vi "Close.vi"(8 "error in":errorcluster, 11 "Climate Chamber in":refnum<class "Climate Chamber.lvclass">) -> (0 "error out":errorcluster, 3 "Climate Chamber out":refnum<class "Climate Chamber.lvclass">)   [LabVIEW 2023, in "Climate Chamber.lvclass"]
uses:
  Climate Chamber.lvclass
  Climate Chamber.lvclass/Climate Chamber.ctl
  Low Level Capabilities/OnOff/OnOff.lvclass
  Low Level Capabilities/Temperature/Temperature Setpoint/Temperature Setpoint.lvclass
  Low Level Capabilities/Temperature/Temperature Actual Value/Temperature Actual Value.lvclass
  Low Level Capabilities/Error/Error.lvclass
  Low Level Capabilities/Temperature/Temperature Gradient/Temperature Gradient.lvclass
  Low Level Capabilities/Temperature/Temperature Limit/Temperature Limit.lvclass
  Low Level Capabilities/Humidity/Humidity Setpoint/Humidity Setpoint.lvclass
  Low Level Capabilities/Humidity/Humidity Limit/Humidity Limit.lvclass
  Low Level Capabilities/Humidity/Humidity Gradient/Humidity Gradient.lvclass
  Low Level Capabilities/Humidity/Humidity Actual Value/Humidity Actual Value.lvclass
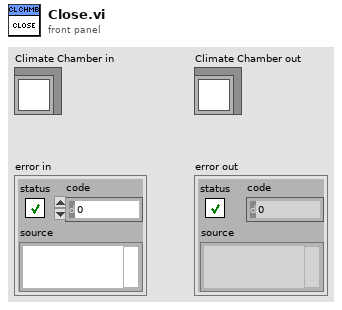
[diagram p1: front panel]
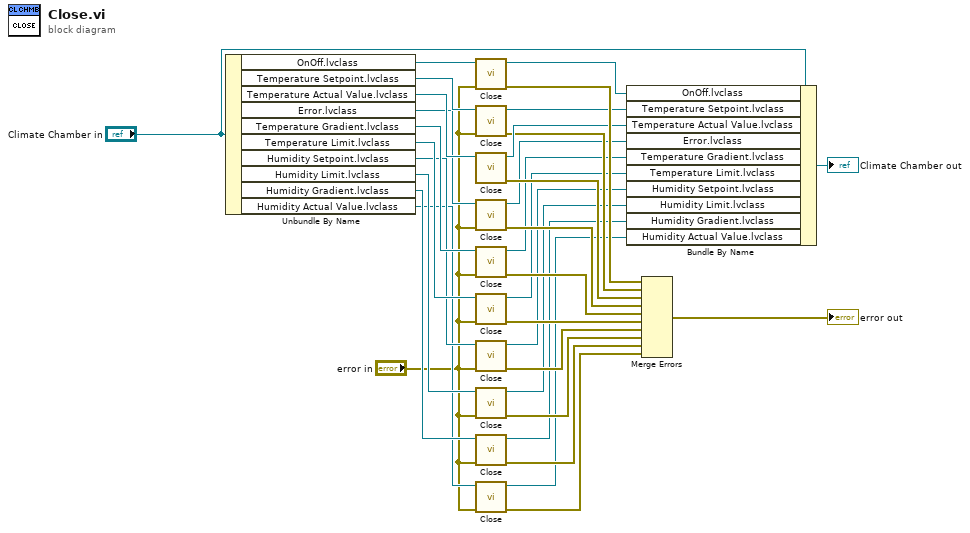
[diagram p0: block diagram]
diagram:
  n1 = Unbundle By Name("Climate Chamber in") -> ("OnOff.lvclass"=w34:refnum<class "OnOff.lvclass">, "Temperature Setpoint.lvclass"=w31:refnum<class "Temperature Setpoint.lvclass">, "Temperature Actual Value.lvclass"=w29:refnum<class "Temperature Actual Value.lvclass">, "Error.lvclass"=w25:refnum<class "Error.lvclass">, "Temperature Gradient.lvclass"=w22:refnum<class "Temperature Gradient.lvclass">, "Temperature Limit.lvclass"=w19:refnum<class "Temperature Limit.lvclass">, "Humidity Setpoint.lvclass"=w16:refnum<class "Humidity Setpoint.lvclass">, "Humidity Limit.lvclass"=w13:refnum<class "Humidity Limit.lvclass">, "Humidity Gradient.lvclass"=w10:refnum<class "Humidity Gradient.lvclass">, "Humidity Actual Value.lvclass"=w7:refnum<class "Humidity Actual Value.lvclass">)
  n2 = call-dynamic "Close.vi"("error in"="error in", "OnOff in"=w34) -> ("error out"=w32:errorcluster, "OnOff out"=w33:refnum<class "OnOff.lvclass">)  [unwired: 8 in]
  n3 = call-dynamic "Close.vi"("error in"="error in", "Temperature Setpoint in"=w31) -> ("error out"=w27:errorcluster, "Temperature Setpoint out"=w30:refnum<class "Temperature Setpoint.lvclass">)  [unwired: 8 in]
  n4 = call-dynamic "Close.vi"("Temperature Actual Value in"=w29) -> ("error out"=w26:errorcluster, "Temperature Actual Value out"=w28:refnum<class "Temperature Actual Value.lvclass">)  [unwired: 9 in]
  n5 = call-dynamic "Close.vi"("error in"="error in", "Error in"=w25) -> ("error out"=w23:errorcluster, "Error out"=w24:refnum<class "Error.lvclass">)  [unwired: 8 in]
  n6 = call-dynamic "Close.vi"("error in"="error in", "Temperature Gradient in"=w22) -> ("error out"=w20:errorcluster, "Temperature Gradient out"=w21:refnum<class "Temperature Gradient.lvclass">)  [unwired: 8 in]
  n7 = call-dynamic "Close.vi"("error in"="error in", "Temperature Limit in"=w19) -> ("error out"=w17:errorcluster, "Temperature Limit out"=w18:refnum<class "Temperature Limit.lvclass">)  [unwired: 8 in]
  n8 = call-dynamic "Close.vi"("error in"="error in", "Humidity Setpoint in"=w16) -> ("error out"=w14:errorcluster, "Humidity Setpoint out"=w15:refnum<class "Humidity Setpoint.lvclass">)  [unwired: 8 in]
  n9 = call-dynamic "Close.vi"("error in"="error in", "Humidity Limit in"=w13) -> ("error out"=w11:errorcluster, "Humidity Limit out"=w12:refnum<class "Humidity Limit.lvclass">)  [unwired: 8 in]
  n10 = call-dynamic "Close.vi"("error in"="error in", "Humidity Gradient in"=w10) -> ("error out"=w8:errorcluster, "Humidity Gradient out"=w9:refnum<class "Humidity Gradient.lvclass">)  [unwired: 8 in]
  n11 = call-dynamic "Close.vi"("error in"="error in", "Humidity Actual Value in"=w7) -> ("error out"=w5:errorcluster, "Humidity Actual Value out"=w6:refnum<class "Humidity Actual Value.lvclass">)  [unwired: 8 in]
  n12 = Bundle By Name(cluster="Climate Chamber in", "OnOff.lvclass"=w33, "Temperature Setpoint.lvclass"=w30, "Temperature Actual Value.lvclass"=w28, "Error.lvclass"=w24, "Temperature Gradient.lvclass"=w21, "Temperature Limit.lvclass"=w18, "Humidity Setpoint.lvclass"=w15, "Humidity Limit.lvclass"=w12, "Humidity Gradient.lvclass"=w9, "Humidity Actual Value.lvclass"=w6) -> (→"Climate Chamber out":refnum<class "Climate Chamber.lvclass">)
  n13 = Merge Errors(w32, w27, w26, w23, w20, w17, w14, w11, w8, w5) -> (→"error out":errorcluster)
